vi "Get Retention Policies.vi"(0 "InfluxDB in":refnum<class "Client.lvclass">, 5 "Database name":string, 11 "error in (no error)":errorcluster) -> (4 "InfluxDB out":refnum<class "Client.lvclass">, 6 "Results Out":refnum<class "Results.lvclass">, 15 "error out":errorcluster)   [LabVIEW 2018, in "InfluxDB Client.lvlib" / "Client.lvclass"]
doc: "Creates a database."
uses:
  Client.lvclass
  Results/Results.lvclass
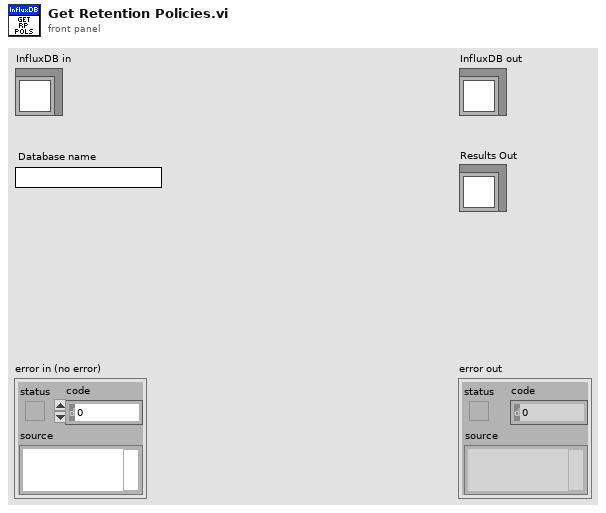
[diagram p1: front panel]
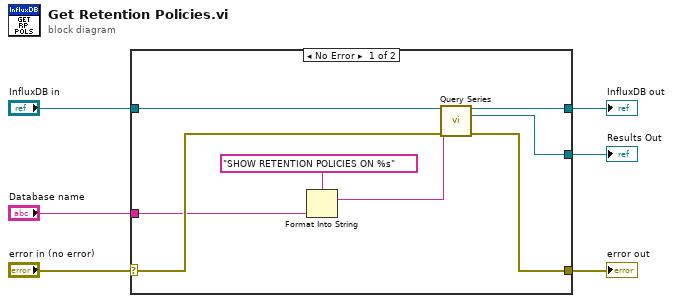
[diagram p0: block diagram]
diagram:
  n1 = case shown="No Error" "error in (no error)" {
    selector: "error in (no error)" -> [w12 w16]
    tunnel: [w10 w16] -> w5
    tunnel: [w13 w15] -> w3
    tunnel: "InfluxDB in" -> [w14 w15]
    tunnel: [w11 _] -> w2
    tunnel: "Database name" -> [w7 _]
    frame No Error {
      n2 = Format Into String(format string="SHOW RETENTION POLICIES ON %s" ("Measurement query"), w7) -> (resulting string=w8:string)  [unwired: 2 in, 1 out]
      n3 = call "Query Series.vi"("InfluxDB in"=w14, "Measurement query"=w8, "error in (no error)"=w12) -> ("InfluxDB out"=w13:refnum<class "Client.lvclass">, "Results Out"=w11:refnum<class "Results.lvclass">, "error out"=w10:errorcluster)  [unwired: 10 in]
    }
    frame Error {
    }
  }
  "error out" <- w5
  "InfluxDB out" <- w3
  "Results Out" <- w2
